vi "Digital Control(RT).vi"() -> ()   [LabVIEW 2013]
uses:
  <vilib>/FPGAPlugInAG/sbRIO-9626/niLvFpga_Open_sbRIO-9626.vi
  <vilib>/rvi/interface/common/dynamic/niFpgaDynamicAddResources.vi
  <vilib>/rvi/interface/common/niFpgaWaitOnOcc.vi
  <vilib>/Utility/error.llb/Error Cluster From Error Code.vi
  <vilib>/rvi/errors/niLvFpgaAdjustHostInterfaceError.vi
  <vilib>/rvi/interface/nirviOpenFPGA/nirviOpenFPGA.xnode
  FPGA/bitfiles/DigitalControl.lvbitx
  <vilib>/rvi/interface/nirviReadWriteControl/nirviReadWriteControl.xnode
  NiFpgaLv.dll
  <vilib>/rvi/interface/Simulation/niFpgaSimulationCallBeginRW.vi
panel:
  in  "Profile":bool
  in  "Profile":dbl[][](array[numeric])
  in  "Pressure":dbl
  in  "RMC/DIO61 (Sol)":bool
  in  "Pos 2 Duty":dbl
  in  "Pos 1 Duty":dbl
  in  "Cycle Frequency":sgl=20.0 min=10 max=200 step=1
  in  "Overlay PWM Frequency":i32=10000 min=20 max=10000 step=1
  in  "HighSide 20Hz PWM overlay":dbl=100.0 min=0.0 max=100.0 step=0.025
  in  "LowSide 20Hz PWM overlay":dbl min=0.0 max=100.0 step=0.025
  in  "Run Condition":T1(ring)=enum."Off"
  in  "20 Hz Duty Cycle":dbl=50.0 min=0.0 max=100.0 step=0.1
  # "cycle freq."
  # "time"
  # "PumpPWM"
  # "20HzDuty"
  # "Pressure"
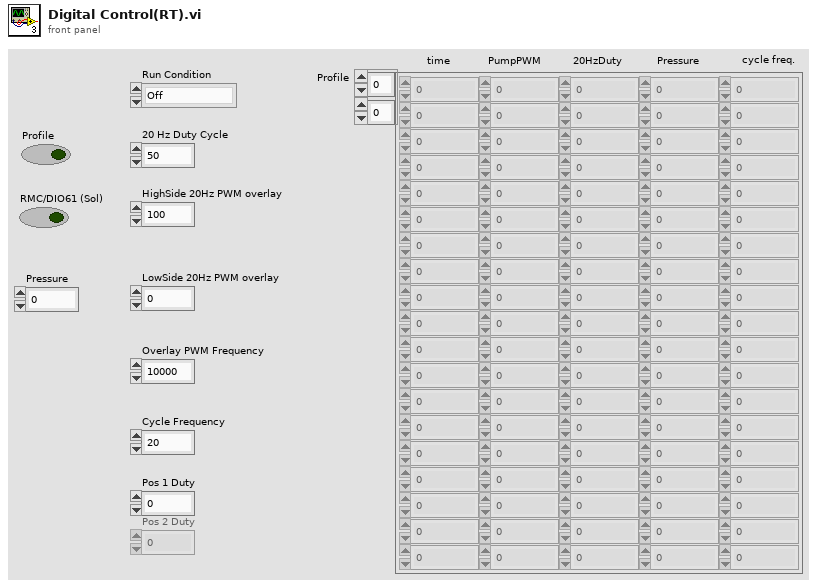
[diagram p1: front panel]
types:
  T1 = enum16{"Cycle", "Low Duty", "High Duty", "On", "Off"}
  T2 = cluster{"Enum":enum16{"Cycle", "Low Duty", "High Duty", "On", "Off"}, "Cycle Duty":dbl, "Duty L":dbl, "Duty H":dbl, "PWM Frequency":i32, "Frequency":sgl, "Pos 1 Duty":dbl, "Pos 2 Duty":dbl, "Pressure":dbl, "RMC/DIO61 (Sol)":bool}
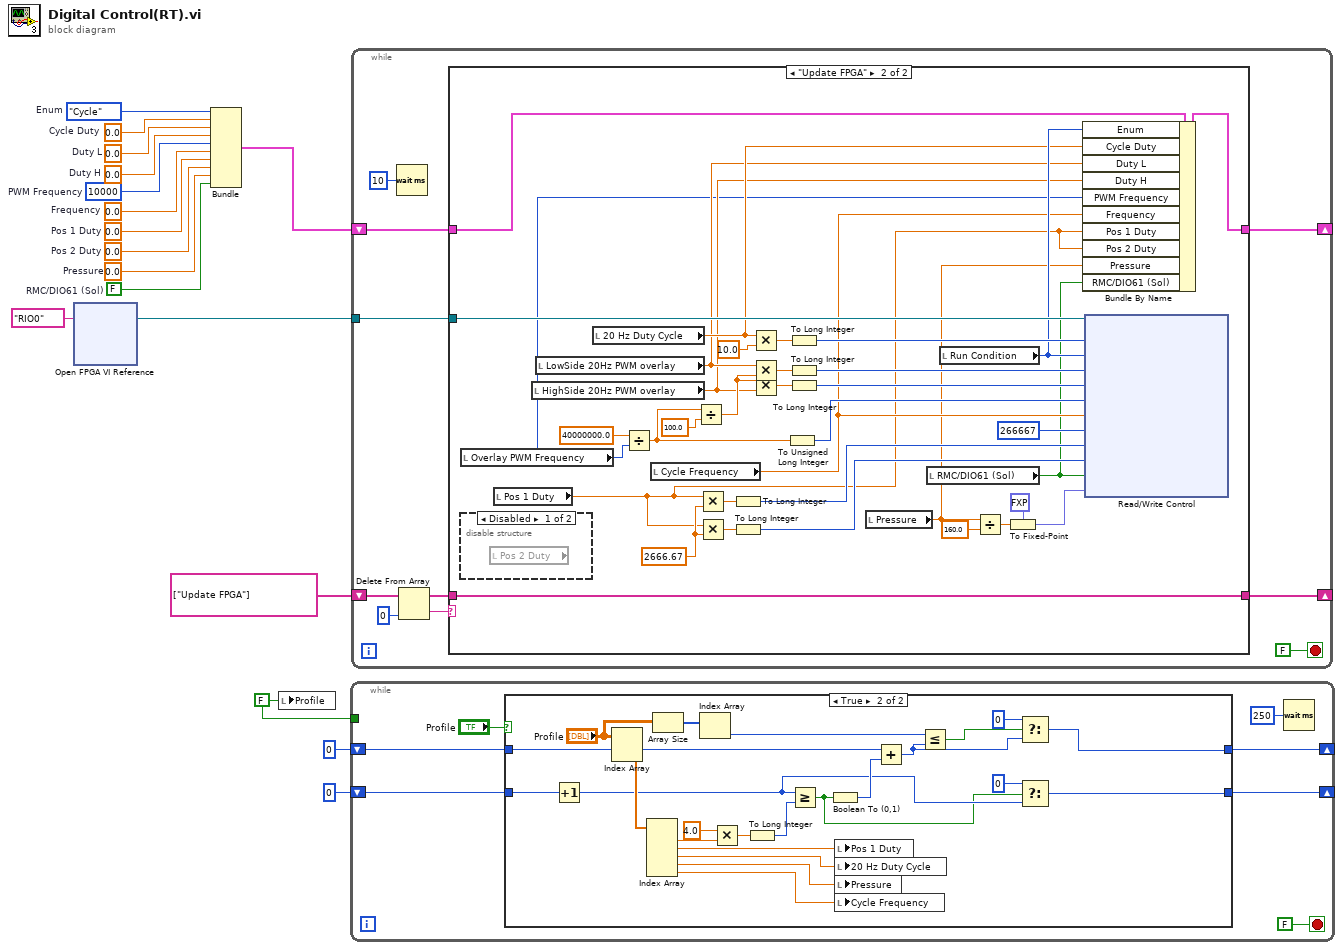
[diagram p0: block diagram]
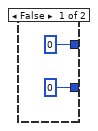
[diagram p2: hidden frame]
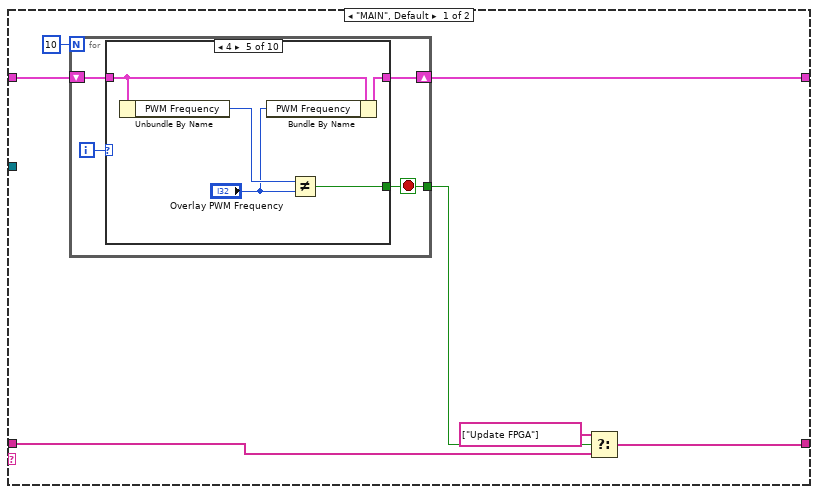
[diagram p3: hidden frame]
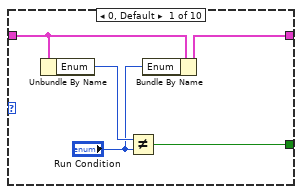
[diagram p4: hidden frame]
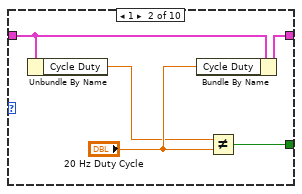
[diagram p5: hidden frame]
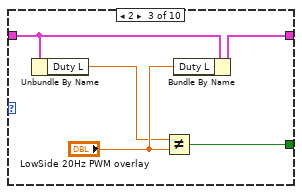
[diagram p6: hidden frame]
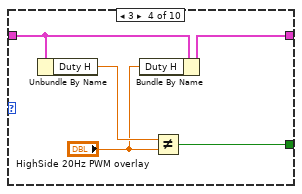
[diagram p7: hidden frame]
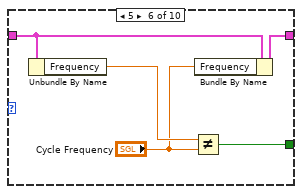
[diagram p8: hidden frame]
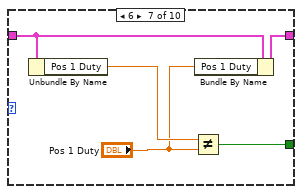
[diagram p9: hidden frame]
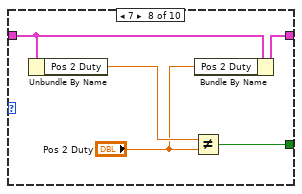
[diagram p10: hidden frame]
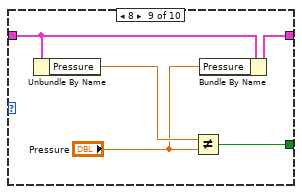
[diagram p11: hidden frame]
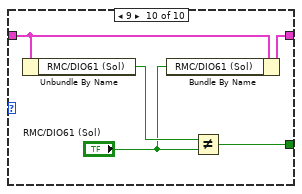
[diagram p12: hidden frame]
diagram:
  w3 = FALSE ("Profile")
  w4 = 10000  # PWM Frequency
  w6 = FALSE  # RMC/DIO61 (Sol)
  w7 = 0.0  # Pressure
  w9 = 0.0  # Pos 1 Duty
  w8 = 0.0  # Pos 2 Duty
  w5 = sgl 0.0  # Frequency
  w11 = 0.0  # Duty H
  w12 = 0.0  # Duty L
  w13 = 0.0  # Cycle Duty
  w14 = T1."Cycle"  # Enum
  n1 = xnode "Open FPGA VI Reference"("resource name"=tag "RIO0") -> ("FPGA VI Reference Out"=w15:refnum<k20>)  [unwired: 1 in, 1 out]
  n2 = Bundle("Enum"=w14, "Cycle Duty"=w13, "Duty L"=w12, "Duty H"=w11, "PWM Frequency"=w4, "Frequency"=w5, "Pos 1 Duty"=w9, "Pos 2 Duty"=w8, "Pressure"=w7, "RMC/DIO61 (Sol)"=w6) -> (w10:T2)  [unwired: 1 in]
  n3 = local write "Profile"(w3) -> ()
  n4 = while {
    tunnel: w3 -> [_]
    shift-right: [w20] -> _
    shift-left: 0 ("index (row)") -> [w21]
    shift-right: [w18] -> _
    shift-left: 0 -> [w19]
    stop <- FALSE stop-if-true
    n5 = case shown="True" "Profile" {
      tunnel: w21 -> [_ w43]
      tunnel: [0 ("index (row)") w32] -> w20
      tunnel: w19 -> [_ w45]
      tunnel: [0 w33] -> w18
      frame False {
      }
      frame True {
        n6 = Increment(x=w45) -> (x+1=w37:i32)
        n7 = Index Array(array="Profile", index (row)=w43) -> (element=w49:dbl[])  [unwired: 1 in]
        n8 = Index Array(array=w49) -> (element #1=w48:dbl, element #2=w31:dbl, element #3=w30:dbl, element #4=w29:dbl, element #5=w27:dbl)  [unwired: 5 in]
        n9 = Array Size(array="Profile") -> (size(s)=w40:i32[])
        n10 = Index Array(array=w40) -> (element=w39:i32)  [unwired: 1 in]
        n11 = Multiply(x=4.0, y=w48) -> (x*y=w46:dbl)
        n12 = To Long Integer(number=w46) -> (32bit integer=w44:i32)
        n13 = Greater Or Equal?(x=w37, y=w44) -> (x >= y?=w28:bool)
        n14 = Boolean To (0,1)(Boolean=w28) -> (0, 1=w42:i16)
        n15 = local write "Pos 1 Duty"(w31) -> ()
        n16 = local write "20 Hz Duty Cycle"(w30) -> ()
        n17 = local write "Pressure"(w29) -> ()
        n18 = local write "Cycle Frequency"(w27) -> ()
        n19 = Add(x=w43, y=w42) -> (x+y=w35:i32)
        n20 = Less Or Equal?(x=w39, y=w35) -> (x <= y?=w38:bool)
        n21 = Select(t=0, s=w38, f=w35) -> (s? t:f=w32:i32)
        n22 = Select(t=0, s=w28, f=w37) -> (s? t:f=w33:i32)
      }
    }
    n23 = Wait (ms)(milliseconds to wait=u32 250) -> ()  [unwired: 1 out]
  }
  n24 = while {
    tunnel: w15 -> [w53]
    shift-right: [w52] -> _
    shift-left: string[] ["Update FPGA"] -> [w57]
    shift-right: [w50] -> _
    shift-left: w10 -> [w51]
    stop <- FALSE stop-if-true
    n25 = Wait (ms)(milliseconds to wait=u32 10) -> ()  [unwired: 1 out]
    n26 = Delete From Array(array=w57, index=0) -> (deleted portion=w54:string, array with subset deleted=w55:string[])  [unwired: 1 in]
    n27 = case shown="\"Update FPGA\"" w54 {
      tunnel: w55 -> [w62 w155]
      tunnel: w53 -> [_ w150]
      tunnel: [w61 w155] -> w52
      tunnel: w51 -> [w64 w131]
      tunnel: [w65 w130] -> w50
      frame "MAIN", Default {
        n28 = for {
          N: 10 -> [_]
          shift-right: [w69] -> w65
          shift-left: w64 -> [w68]
          tunnel: [w67] -> w63
          i -> [w70]
          stop <- w67 stop-if-true
          n29 = case shown="4" w70 {
            tunnel: w68 -> [w75 w80 w85 w90 w95 w100 w105 w110 w115 w120]
            tunnel: [w74 w79 w84 w89 w94 w99 w104 w109 w114 w119] -> w69
            tunnel: [w71 w76 w81 w88 w93 w98 w103 w108 w113 w118] -> w67
            frame 0, Default {
              n30 = Unbundle By Name(w75) -> ("Enum"=w73:T1)
              n31 = Not Equal?(x=w73, y="Run Condition") -> (x != y?=w71:bool)
              n32 = Bundle By Name(cluster=w75, "Enum"="Run Condition") -> (w74:T2)
            }
            frame 1 {
              n33 = Unbundle By Name(w80) -> ("Cycle Duty"=w77:dbl)
              n34 = Bundle By Name(cluster=w80, "Cycle Duty"="20 Hz Duty Cycle") -> (w79:T2)
              n35 = Not Equal?(x=w77, y="20 Hz Duty Cycle") -> (x != y?=w76:bool)
            }
            frame 2 {
              n36 = Unbundle By Name(w85) -> ("Duty L"=w82:dbl)
              n37 = Not Equal?(x=w82, y="LowSide 20Hz PWM overlay") -> (x != y?=w81:bool)
              n38 = Bundle By Name(cluster=w85, "Duty L"="LowSide 20Hz PWM overlay") -> (w84:T2)
            }
            frame 3 {
              n39 = Unbundle By Name(w90) -> ("Duty H"=w87:dbl)
              n40 = Bundle By Name(cluster=w90, "Duty H"="HighSide 20Hz PWM overlay") -> (w89:T2)
              n41 = Not Equal?(x=w87, y="HighSide 20Hz PWM overlay") -> (x != y?=w88:bool)
            }
            frame 4 {
              n42 = Unbundle By Name(w95) -> ("PWM Frequency"=w92:i32)
              n43 = Bundle By Name(cluster=w95, "PWM Frequency"="Overlay PWM Frequency") -> (w94:T2)
              n44 = Not Equal?(x=w92, y="Overlay PWM Frequency") -> (x != y?=w93:bool)
            }
            frame 5 {
              n45 = Unbundle By Name(w100) -> ("Frequency"=w97:sgl)
              n46 = Not Equal?(x=w97, y="Cycle Frequency") -> (x != y?=w98:bool)
              n47 = Bundle By Name(cluster=w100, "Frequency"="Cycle Frequency") -> (w99:T2)
            }
            frame 6 {
              n48 = Unbundle By Name(w105) -> ("Pos 1 Duty"=w102:dbl)
              n49 = Not Equal?(x=w102, y="Pos 1 Duty") -> (x != y?=w103:bool)
              n50 = Bundle By Name(cluster=w105, "Pos 1 Duty"="Pos 1 Duty") -> (w104:T2)
            }
            frame 7 {
              n51 = Unbundle By Name(w110) -> ("Pos 2 Duty"=w107:dbl)
              n52 = Not Equal?(x=w107, y="Pos 2 Duty") -> (x != y?=w108:bool)
              n53 = Bundle By Name(cluster=w110, "Pos 2 Duty"="Pos 2 Duty") -> (w109:T2)
            }
            frame 8 {
              n54 = Unbundle By Name(w115) -> ("Pressure"=w112:dbl)
              n55 = Not Equal?(x=w112, y="Pressure") -> (x != y?=w113:bool)
              n56 = Bundle By Name(cluster=w115, "Pressure"="Pressure") -> (w114:T2)
            }
            frame 9 {
              n57 = Unbundle By Name(w120) -> ("RMC/DIO61 (Sol)"=w117:bool)
              n58 = Bundle By Name(cluster=w120, "RMC/DIO61 (Sol)"="RMC/DIO61 (Sol)") -> (w119:T2)
              n59 = Not Equal?(x=w117, y="RMC/DIO61 (Sol)") -> (x != y?=w118:bool)
            }
          }
        }
        n60 = Select(t=string[] ["Update FPGA"], s=w63, f=w62) -> (s? t:f=w61:string[])
      }
      frame "Update FPGA" {
        w139 = 2666.67
        n61 = local read "Overlay PWM Frequency"() -> (w125:i32)
        n62 = disable-structure shown="Disabled" {
          frame Disabled {
            n63 = local read "Pos 2 Duty"() -> ()  [unwired: 1 out]
          }
          frame Enabled {
          }
        }
        n64 = local read "Pos 1 Duty"() -> (w123:dbl)
        n65 = local read "HighSide 20Hz PWM overlay"() -> (w126:dbl)
        n66 = local read "LowSide 20Hz PWM overlay"() -> (w127:dbl)
        n67 = local read "20 Hz Duty Cycle"() -> (w128:dbl)
        n68 = Divide(x=40000000.0, y=w125) -> (x/y=w144:dbl)
        n69 = local read "Cycle Frequency"() -> (w124:sgl)
        n70 = Divide(x=w144, y=100.0) -> (x/y=w132:dbl)
        n71 = Multiply(x=w123, y=w139) -> (x*y=w141:dbl)
        n72 = Multiply(x=w123, y=w139) -> (x*y=w140:dbl)
        n73 = To Long Integer(number=w141) -> (32bit integer=w138:i32)
        n74 = To Long Integer(number=w140) -> (32bit integer=w137:i32)
        n75 = Multiply(x=w128, y=10.0) -> (x*y=w153:dbl)
        n76 = Multiply(x=w127, y=w132) -> (x*y=w152:dbl)
        n77 = Multiply(x=w132, y=w126) -> (x*y=w151:dbl)
        n78 = To Unsigned Long Integer(number=w144) -> (unsigned 32bit integer=w145:u32)
        n79 = To Long Integer(number=w153) -> (32bit integer=w149:i32)
        n80 = To Long Integer(number=w152) -> (32bit integer=w148:i32)
        n81 = To Long Integer(number=w151) -> (32bit integer=w147:i32)
        n82 = local read "Pressure"() -> (w122:dbl)
        n83 = local read "RMC/DIO61 (Sol)"() -> (w121:bool)
        n84 = local read "Run Condition"() -> (w129:T1)
        n85 = Divide(x=w122, y=160.0) -> (x/y=w136:dbl)
        n86 = To Fixed-Point(fixed-point type=fxp<+/-,20,5> 0.0 ("AO0"), number=w136) -> (fixed-point=w133:fxp<+/-,20,5>)
        n87 = Bundle By Name(cluster=w131, "Enum"=w129, "Cycle Duty"=w128, "Duty L"=w127, "Duty H"=w126, "PWM Frequency"=w125, "Frequency"=w124, "Pos 1 Duty"=w123, "Pos 2 Duty"=w123, "Pressure"=w122, "RMC/DIO61 (Sol)"=w121) -> (w130:T2)
        n88 = xnode "Read/Write Control"("FPGA VI Reference In"=w150, "Cycle Duty"=w149, "Enum"=w129, "Duty L"=w148, "Duty H"=w147, "PWM Period"=w145, "Frequency"=w124, "Controller Period (ticks)"=u32 266667, "Duty 1 (Ticks)"=w138, "Duty 2 (Ticks)"=w137, "RMC/DIO61"=w121, "AO0"=w133) -> ()  [unwired: 1 in, 2 out]
      }
    }
  }
